vi "InitializeVersion.vi"(7 "Action":T1, 8 "error in (no error)":errorcluster, 10 "Application":refnum<vi>, 11 "LVClass ref":refnum<vi>) -> (0 "error out":errorcluster, 1 "BlueSerializableVersion":u16, 2 "Application":refnum<vi>, 3 "LVClass ref":refnum<vi>)   [LabVIEW 2019, in "BlueSerializationScripts.lvlib"]
uses:
  BlueSerializationScripts.lvlib
  UserAppLibs/IncrementMutationHistory/IncrementBlueSerVersionAction.ctl
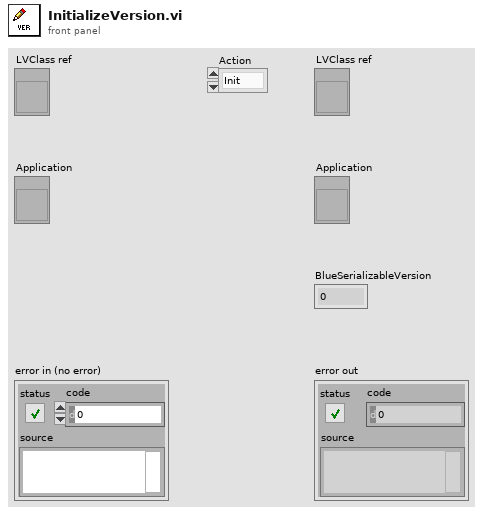
[diagram p1: front panel]
types:
  T1 = typedef "BlueSerializationScripts.lvlib/IncrementBlueSerVersionAction.ctl" = enum16{"Init", "Increment"}
  T2 = cluster{"Major":u16, "Minor":u16, "Fix":u16, "Build":u16}
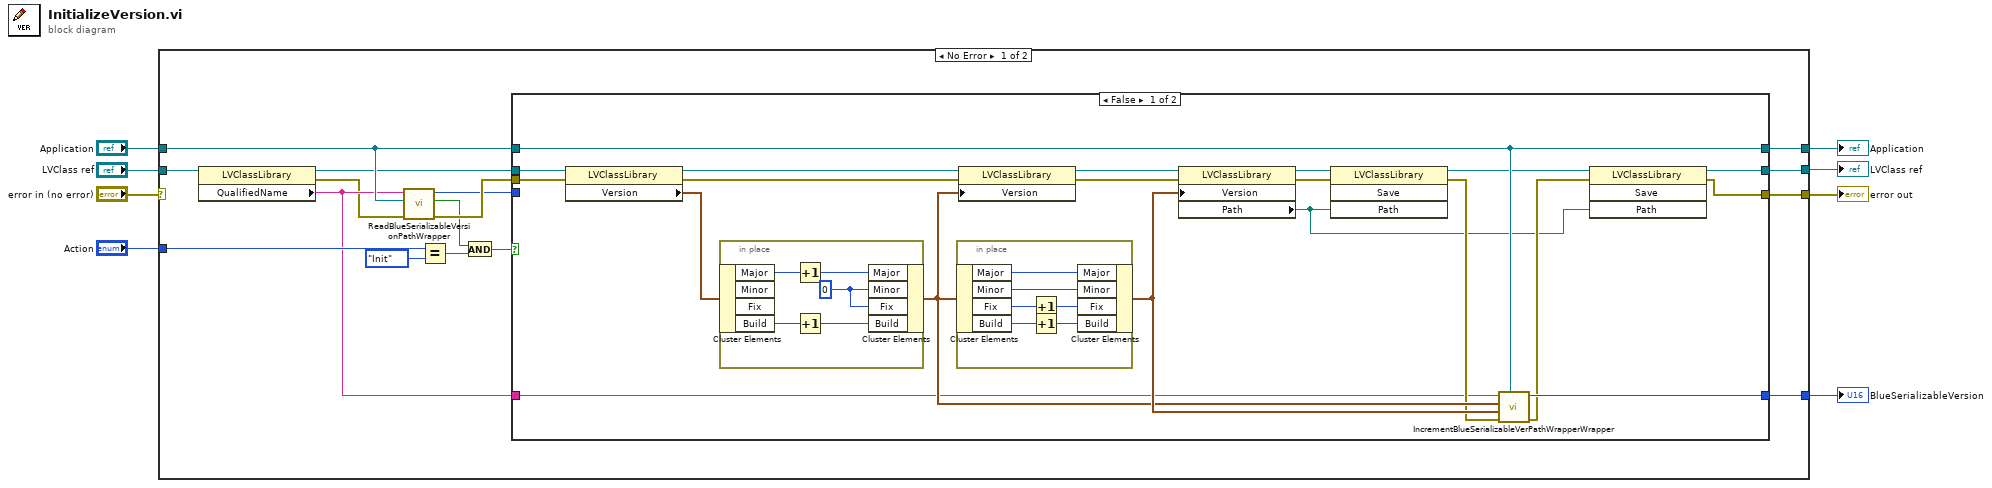
[diagram p0: block diagram]
diagram:
  n1 = case shown="No Error" "error in (no error)" {
    selector: "error in (no error)" -> [_ w62]
    tunnel: [w24 w62] -> w8
    tunnel: [w23 w61] -> w7
    tunnel: "Application" -> [w17 w61]
    tunnel: "Action" -> [w22 _]
    tunnel: [w18 _] -> w3
    tunnel: "LVClass ref" -> [w15 w60]
    tunnel: [w11 w60] -> w1
    frame No Error {
      n2 = property class="LVClassLibrary"(reference=w15) -> (reference out=w13:refnum<vi>, error out=w12:errorcluster, "QualifiedName"=w14:string)  [unwired: 1 in]
      n3 = call "ReadBlueSerializableVersionPathWrapper.vi"("error in (no error)"=w12, "Application"=w17, "LVClass name"=w14) -> ("error out"=w16:errorcluster, "BlueSerializableVersion found?"=w10:bool, "BlueSerializableVersion"=w9:u16)  [unwired: 6 in]
      n4 = Equal?(x=w22, y=IncrementBlueSerVersionAction."Init") -> (x = y?=w20:bool)
      n5 = And(x=w10, y=w20) -> (x .and. y?=w19:bool)
      n6 = case shown="False" w19 {
        tunnel: w16 -> [w44 w59]
        tunnel: [w26 w59] -> w24
        tunnel: w17 -> [w43 w58]
        tunnel: [w43 w58] -> w23
        tunnel: [w33 w56] -> w18
        tunnel: w13 -> [w31 w57]
        tunnel: w14 -> [w28 _]
        tunnel: [w25 w57] -> w11
        tunnel: w9 -> [_ w56]
        frame False {
          n7 = property class="LVClassLibrary"(reference=w31, error in=w44) -> (reference out=w41:refnum<vi>, error out=w40:errorcluster, "Version"=w42:T2)
          n8 = in-place {
            w47 = u16 0 ("Library Version.Minor")
            n9 = in-place-cluster #1(w42) -> ("Major"=w49:u16, "Build"=w46:u16)  [unwired: 2 out]
            n10 = Increment(x=w49) -> (x+1=w48:u16)
            n11 = Increment(x=w46) -> (x+1=w45:u16)
            n12 = in-place-cluster #1("Major"=w48, "Minor"=w47, "Fix"=w47, "Build"=w45) -> (w34:T2)
          }
          n13 = in-place {
            n14 = in-place-cluster #2(w34) -> ("Major"=w50:u16, "Minor"=w51:u16, "Fix"=w53:u16, "Build"=w55:u16)
            n15 = Increment(x=w53) -> (x+1=w52:u16)
            n16 = Increment(x=w55) -> (x+1=w54:u16)
            n17 = in-place-cluster #2("Major"=w50, "Minor"=w51, "Fix"=w52, "Build"=w54) -> (w35:T2)
          }
          n18 = property class="LVClassLibrary"(reference=w41, error in=w40, "Version"=w34) -> (reference out=w39:refnum<vi>, error out=w38:errorcluster)
          n19 = property class="LVClassLibrary"(reference=w39, error in=w38, "Version"=w35) -> (reference out=w37:refnum<vi>, error out=w36:errorcluster, "Path"=w27:path)
          n20 = invoke class="LVClassLibrary" method="Save"(reference=w37, error in=w36, "Path"=w27) -> (reference out=w29:refnum<vi>, error out=w30:errorcluster)  [unwired: 1 in, 2 out]
          n21 = call "IncrementBlueSerializableVerPathWrapperWrapper.vi"("Application"=w43, "error in (no error)"=w30, "Version Bump 2"=w35, "Version Bump 1"=w34, "LVClass name"=w28) -> ("error out"=w32:errorcluster, "BlueSerializableVersion"=w33:u16)  [unwired: 5 in]
          n22 = invoke class="LVClassLibrary" method="Save"(reference=w29, error in=w32, "Path"=w27) -> (reference out=w25:refnum<vi>, error out=w26:errorcluster)  [unwired: 1 in, 2 out]
        }
        frame True {
        }
      }
    }
    frame Error {
    }
  }
  "error out" <- w8
  "Application" <- w7
  "BlueSerializableVersion" <- w3
  "LVClass ref" <- w1
